vi "KH7008 COM.vi"(2 "error in (no error)":errorcluster, 3 "Command":string, 4 "VISA Refnum in":refnum<visa-resource-name>="COM3") -> (0 "error out":errorcluster, 1 "Response":string="\r\n")   [LabVIEW 2013]
uses:
  <vilib>/Instr/_visa.llb/VISA Configure Serial Port (Instr).vi
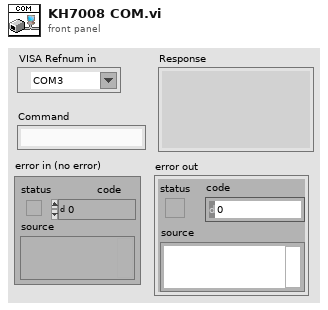
[diagram p1: front panel]
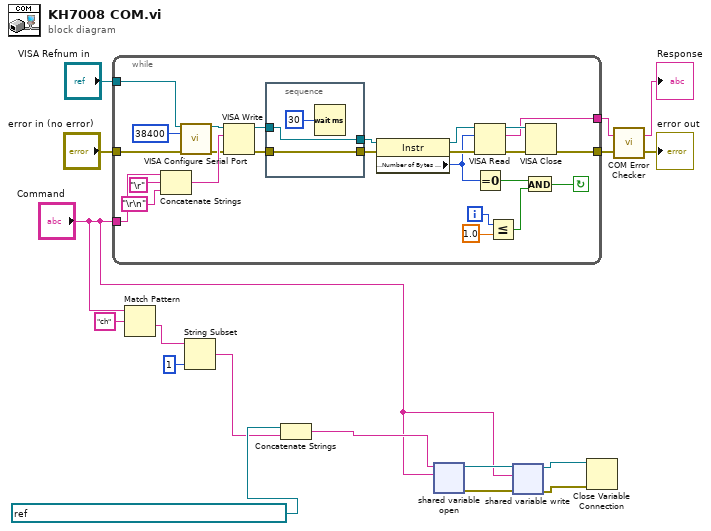
[diagram p0: block diagram]
diagram:
  n1 = while {
    tunnel: "VISA Refnum in" -> [w28]
    tunnel: "Command" -> [w27]
    tunnel: "error in (no error)" -> [w20]
    tunnel: [w19] -> w14
    tunnel: [w18] -> w15
    i -> [w24]
    stop <- w21 continue-if-true
    n2 = Concatenate Strings(w27, "\r", "\r\n") -> (w42:string)
    n3 = call-poly "VISA Configure Serial Port"("VISA resource name"=w28, "baud rate (9600)"=u32 38400 ("baud rate"), "error in (no error)"=w20) -> ("VISA resource name out"=w38:refnum<visa-resource-name>, "error out"=w39:errorcluster)  [unwired: 6 in, 5 out]
    n4 = VISA Write(VISA resource name=w38, write buffer=w42, error in (no error)=w39) -> (VISA resource name out=w34:refnum<visa-resource-name>, error out=w32:errorcluster)  [unwired: 1 out]
    n5 = stacked-sequence {
      tunnel: w32 -> [w45]
      tunnel: [w45] -> w33
      tunnel: w34 -> [w44]
      tunnel: [w44] -> w35
      frame #0 {
        n6 = Wait (ms)(milliseconds to wait=u32 30) -> ()  [unwired: 1 out]
      }
    }
    n7 = property class="Instr"(reference=w35, error in=w33) -> (reference out=w36:refnum<visa-resource-name>, error out=w37:errorcluster, "Serial Settings:Number of Bytes at Serial Port"=w26:u32)
    n8 = VISA Read(VISA resource name=w36, byte count=w26, error in (no error)=w37) -> (VISA resource name out=w31:refnum<visa-resource-name>, read buffer=w18:string, error out=w30:errorcluster)  [unwired: 1 out]
    n9 = Equal To 0?(x=w26) -> (x = 0?=w23:bool)
    n10 = Less Or Equal?(x=w24, y=1.0) -> (x <= y?=w22:bool)
    n11 = And(x=w23, y=w22) -> (x .and. y?=w21:bool)
    n12 = VISA Close(VISA resource name=w31, error in (no error)=w30) -> (error out=w19:errorcluster)
  }
  n13 = Match Pattern(string="Command", regular expression="ch") -> (after substring=w10:string)  [unwired: 1 in, 3 out]
  n14 = String Subset(string=w10, length (rest)=1 ("length (rest)")) -> (substring=w3:string)  [unwired: 1 in]
  n15 = Concatenate Strings(refnum<k21> "ni.var.psp://housesoftheholy/MNK_18T/KH_ch" ("shared variable refnum in"), w3) -> (w2:string)
  n16 = shared-variable-open(w2, "Command") -> (w8:refnum<k21>, w6:errorcluster)  [unwired: 2 in]
  n17 = shared-variable-write(w8, w6, "Command") -> (w7:refnum<k21>, w5:errorcluster)
  n18 = Close Variable Connection(8:w5, 11:w7) -> ()  [unwired: 1 out]
  n19 = call "COM Error Checker.vi"("error in (no error)"=w14, "String In"=w15) -> ("error out"=→"error out":errorcluster, "String"=→"Response":string)
